vi "Cramer SoS.vi"(9 "Atmospheric pressure in Pa":dbl=101325.0, 10 "Temperature":dbl, 11 "Humidity":dbl=60.0) -> (3 "Cramer SoS":dbl format="%#_8g")   [LabVIEW 2018]
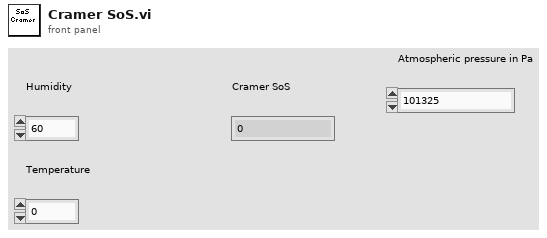
[diagram p1: front panel]
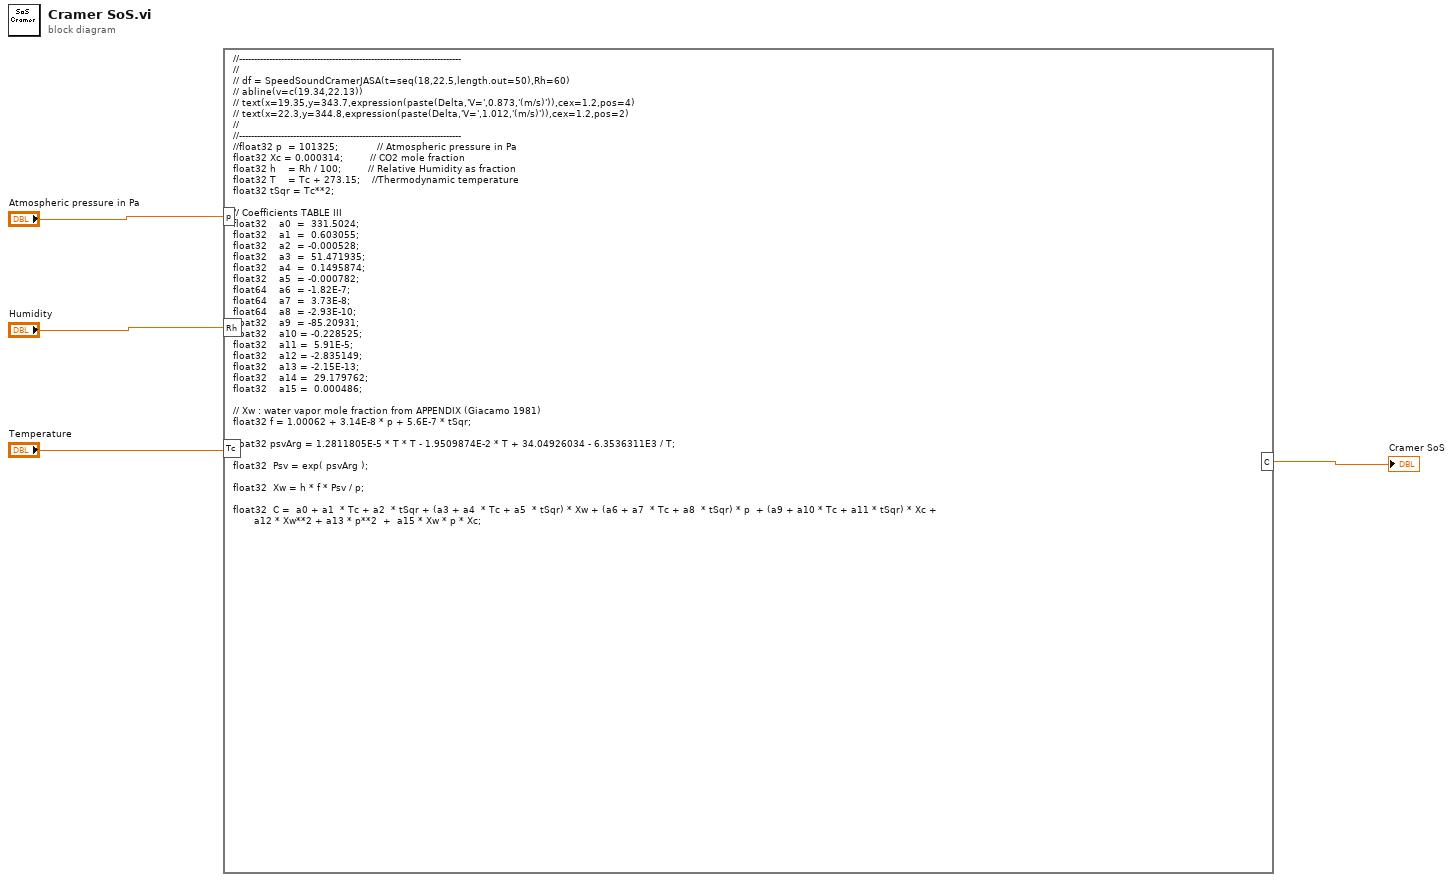
[diagram p0: block diagram]
diagram:
  n1 = formula code="//--------------------------------------------------------------------------\n//\n// df = SpeedSoundCramerJASA(t=seq(18,22.5,length.out=50),Rh=60)\n// abline(v=c(19.34,22.13))\n// text(x=19.35,y=343.7,expression(paste(Delta,'V=',0.873,'(m/s)')),cex=1.2,pos=4)\n// text(x=22.3,y=344.8,expression(paste(Delta,'V=',1.012,'(m/s)')),cex=1.2,pos=2)\n//\n//--------------------------------------------------------------------------\n//float32 p  = 101325;             // Atmospheric pressure in Pa\nfloat32 Xc = 0.000314;         // CO2 mole fraction\nfloat32 h    = Rh / 100;         // Relative Humidity as fraction\nfloat32 T    = Tc + 273.15;    //Thermodynamic temperature\nfloat32 tSqr = Tc**2;\n\n// Coefficients TABLE III\nfloat32    a0  =  331.5024;\nfloat32    a1  =  0.603055;\nfloat32    a2  = -0.000528;\nfloat32    a3  =  51.471935;\nfloat32    a4  =  0.1495874;\nfloat32    a5  = -0.000782;\nfloat64    a6  = -1.82E-7;\nfloat64    a7  =  3.73E-8;\nfloat64    a8  = -2.93E-10;\nfloat32    a9  = -85.20931;\nfloat32    a10 = -0.228525;\nfloat32    a11 =  5.91E-5;\nfloat32    a12 = -2.835149;\nfloat32    a13 = -2.15E-13;\nfloat32    a14 =  29.179762;\nfloat32    a15 =  0.000486;\n\n// Xw : water vapor mole fraction from APPENDIX (Giacamo 1981)\nfloat32 f = 1.00062 + 3.14E-8 * p + 5.6E-7 * tSqr;\n\nfloat32 psvArg = 1.2811805E-5 * T * T - 1.9509874E-2 * T + 34.04926034 - 6.3536311E3 / T;\n\nfloat32  Psv = exp( psvArg );\n\nfloat32  Xw = h * f * Psv / p;\n\nfloat32  C =  a0 + a1  * Tc + a2  * tSqr + (a3 + a4  * Tc + a5  * tSqr) * Xw + (a6 + a7  * Tc + a8  * tSqr) * p  + (a9 + a10 * Tc + a11 * tSqr) * Xc +\n       a12 * Xw**2 + a13 * p**2  +  a15 * Xw * p * Xc;"("Tc"="Temperature", "Rh"="Humidity", "p"="Atmospheric pressure in Pa") -> ("C"=→"Cramer SoS":sgl)
